vi "Subarray Lorentz fit 1.vi"(6 "cursor diff":dbl, 9 "cursor avg":dbl, 10 "Y subset":dbl[](array[numeric]), 11 "X subset":dbl[](array[numeric])) -> (0 "error out":errorcluster, 1 "Initial params":dbl[](array[numeric]), 2 "best fit parameters":dbl[](array[numeric]), 3 "best nonlinear fit":dbl[](array[numeric]))   [LabVIEW 2015]
uses:
  <vilib>/gmath/NumericalOptimization/Nonlinear Curve Fit LM bound.vi
  <vilib>/gmath/NI_Gmath.lvlib
panel:
  # "Fitting to an actual Lorentzian: only two free parameters"
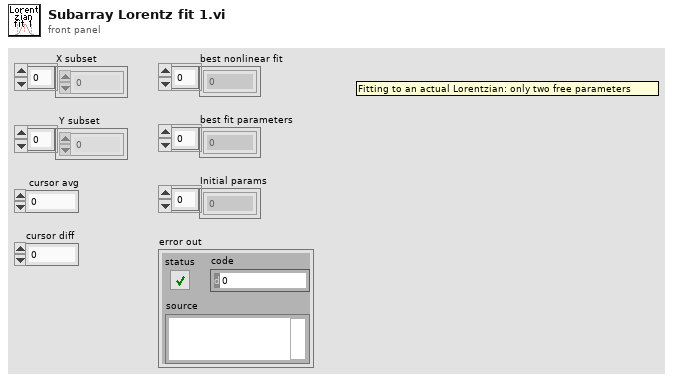
[diagram p1: front panel]
types:
  T1 = cluster{"parameter minimum":dbl[], "parameter maximum":dbl[]}
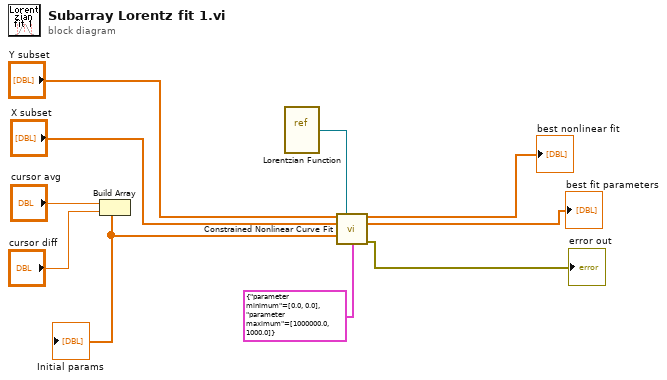
[diagram p0: block diagram]
diagram:
  n1 = Build Array("cursor avg", "cursor diff") -> (w1:dbl[])
  "Initial params" <- w1
  n2 = vi-ref "Lorentzian Function.vi"() -> (w10:refnum<vi>)
  n3 = call-poly <vilib>:"Constrained Nonlinear Curve Fit.vi"("Y"="Y subset", "f(x,a)"=w10, "X"="X subset", "initial parameters"=w1, "parameter bounds"=T1 {"parameter minimum"=[0.0, 0.0], "parameter maximum"=[1000000.0, 1000.0]}) -> ("best nonlinear fit"=→"best nonlinear fit":dbl[], "best fit parameters"=→"best fit parameters":dbl[], "error out"=→"error out":errorcluster)  [unwired: 5 in, 3 out]
